vi "HRV_main.vi"() -> ()   [LabVIEW 2009]
uses:
  Instance           4 13Saved   HRV_3 .vi
  Instance           3 13Saved   HRV_3 .vi
  Instance           2 13Saved   HRV_3 .vi
  Instance           1 13Saved   HRV_3 .vi
  Instance           5 13Saved   HRV_3 .vi
  Instance           6 13Saved   HRV_3 .vi
  Instance           7 13Saved   HRV_3 .vi
  Instance           9 13Saved   HRV_3 .vi
  <vilib>/Analysis/5stat.llb/RMS (DBL).vi
  Instance          21 13Saved   HRV_3 .vi
  Instance          20 13Saved   HRV_3 .vi
  Instance          19 13Saved   HRV_3 .vi
  Instance          24 13Saved   HRV_3 .vi
  Instance          23 13Saved   HRV_3 .vi
  Instance          22 13Saved   HRV_3 .vi
  Instance          18 13Saved   HRV_3 .vi
  Instance          17 13Saved   HRV_3 .vi
  Instance          16 13Saved   HRV_3 .vi
  Instance          14 13Saved   HRV_3 .vi
  Instance          13 13Saved   HRV_3 .vi
  <vilib>/express/express analysis/Spectral/XNode/ExpressSpectralMeasurementsBlockNode.xnode
  <vilib>/express/express analysis/Spectral/Block/exnSpectralBlock spectral measurements PSD poly.vi
  <vilib>/express/express analysis/Spectral/Block/exnSpectralBlock spectral measurements PSD DDT.vi
  Instance          25 13Saved   HRV_3 .vi
  Instance          26 13Saved   HRV_3 .vi
  Instance          27 13Saved   HRV_3 .vi
  <vilib>/Utility/NIReport.llb/HTML Report Text Alignment.ctl
  <vilib>/Utility/NIReport.llb/NI_report.lvclass
  <vilib>/printing/OpenHTMLReport.llb/Open HTML Report in Browser (Refnum).vi
  <vilib>/Utility/NIReport.llb/Append Report Text (str wrap).vi
  <vilib>/Analysis/NI_AALPro.lvlib
  <vilib>/Analysis/NI_AALBase.lvlib
  <vilib>/Utility/NIReport.llb/NI_ReportGenerationCore.lvlib
panel:
  out "Waveform Graph":dynamicdata(graph)
  out "File Name:":string
  in  "Sample Rate:":sgl=500.034 min=1 max=20000 format="%.3g"
  in  "Tab Control 3":enum32{"RR-Intervals", "HRV"}(tab)=enum."HRV"
  in  "RR Rejection  Sensitivity :":dbl=0.5 min=0.0 max=1.0 format="%#.5g"
  in  "Resample Rate : (Hz):":dbl=2.0 format="%.3p"
  out "RR Waveforms":dbl[][](graph)
  out "HRV: Freq Domain":string[][](table)
  in  "HF2":dbl=0.4 caption="Begin Offset" min=0.0
  in  "HF1":dbl=0.15 caption="Begin Offset" min=0.0
  in  "LF2":dbl=0.15 caption="Begin Offset" min=0.0
  in  "LF1":dbl=0.04 caption="Begin Offset" min=0.0
  in  "TP 2":dbl=0.4 caption="Begin Offset" min=0.0
  in  "TP 1":dbl=0.04 caption="Begin Offset" min=0.0
  out "HRV: Time Domain":string[][](table)
  out "RR FFT 2":dynamicdata(graph) caption="Power Spectrum"
  out "ECG Waveform":dbl[][](graph)
  in  "Tab Control":enum32{"Controls", "Filters"}(tab)
  in  "File Type":u16(ring) items=["ASCII (*.txt)", "Binary (*.tdx)"]
  in  "Report Type":enum16{"Standard Report", "HTML"}(ring)=enum."HTML"
  in  "Save :":bool
  in  "Save RR data to file:":bool
  in  "Threshold:":dbl=1.0 step=0.001 format="%#.6f"
  out "Number of Peaks:":i32
  in  "Select ECG":bool
  in  "Report":bool
  in  "Bandstop":bool=TRUE
  in  "Lower Cut-Off":dbl=59.0 format="%#_4g"
  in  "Upper Cut-Off":dbl=61.0 format="%#_4g"
  in  "Bandpass":bool=TRUE
  in  "Upper Cut-Off":dbl=100.0 format="%#_4g"
  in  "Lower Cut-Off":dbl=0.05 format="%#_4g"
  # "Frequency Domain"
  # "Frequency Limits"
  # "LF Limits:"
  # "HF Limits:"
  # "Total Limits:"
  # "Time Domain"
  # "Bandpass"
  # "Bandstop"
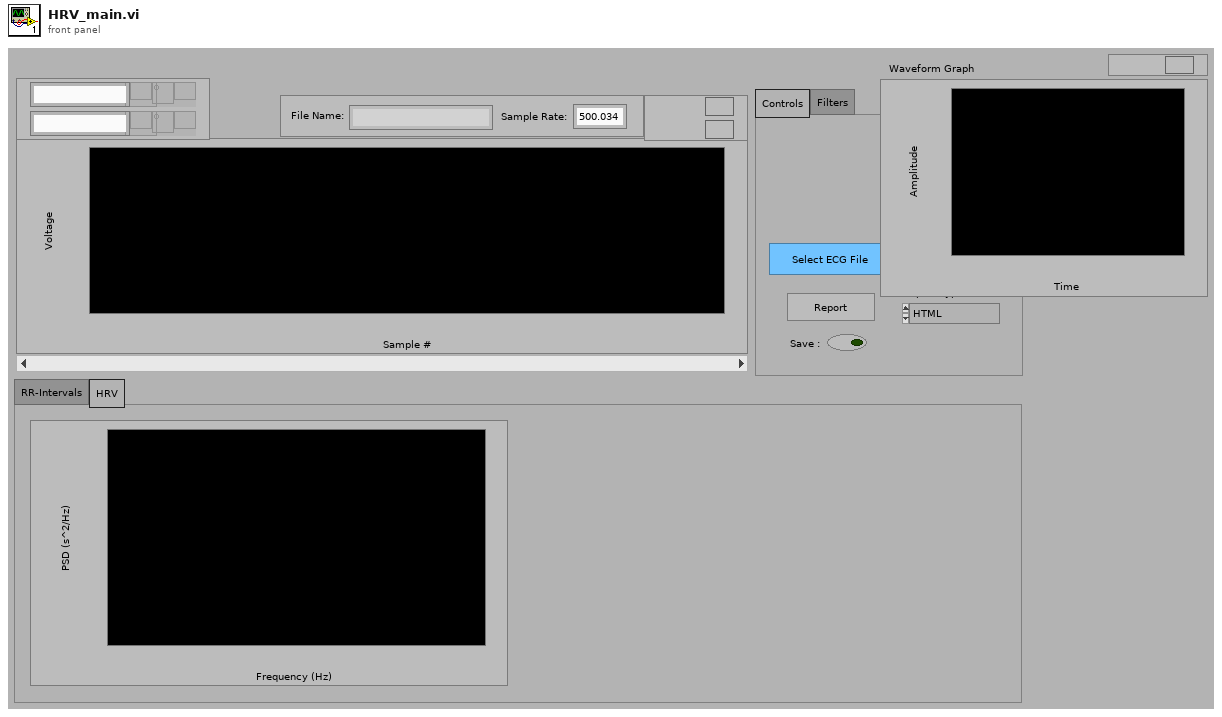
[diagram p1: front panel]
types:
  T1 = cluster{"averaging mode":u16, "weighting mode":u16, "number of averages":u32}
  T2 = cluster{"dB On (F)":bool, "unwrap phase (F)":bool, "convert to degree (F)":bool}
  T3 = typedef "NI_ReportGenerationCore.lvlib/HTML Report Text Alignment.ctl" = enum16{"(default)", "LEFT", "CENTER", "RIGHT"}
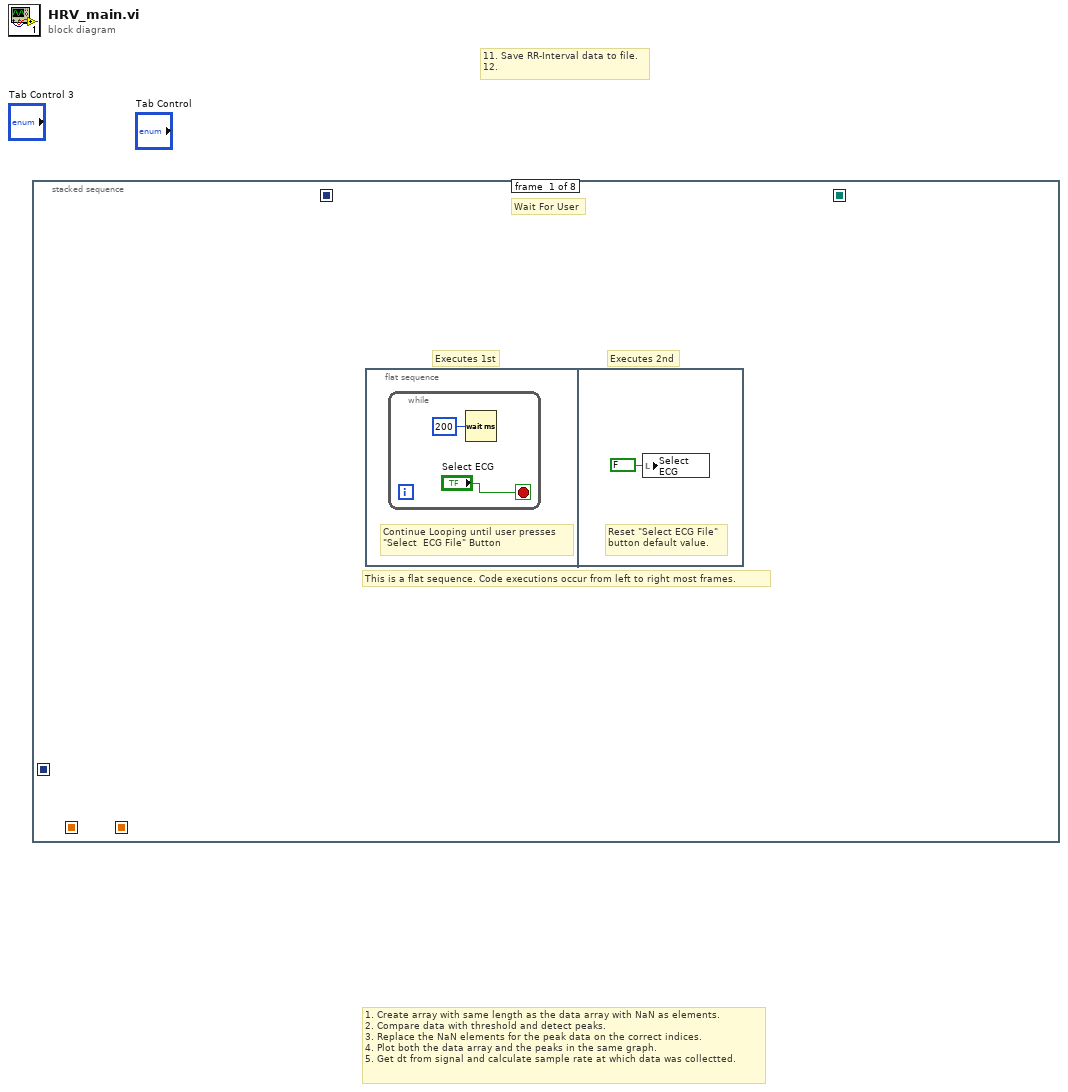
[diagram p0: block diagram]
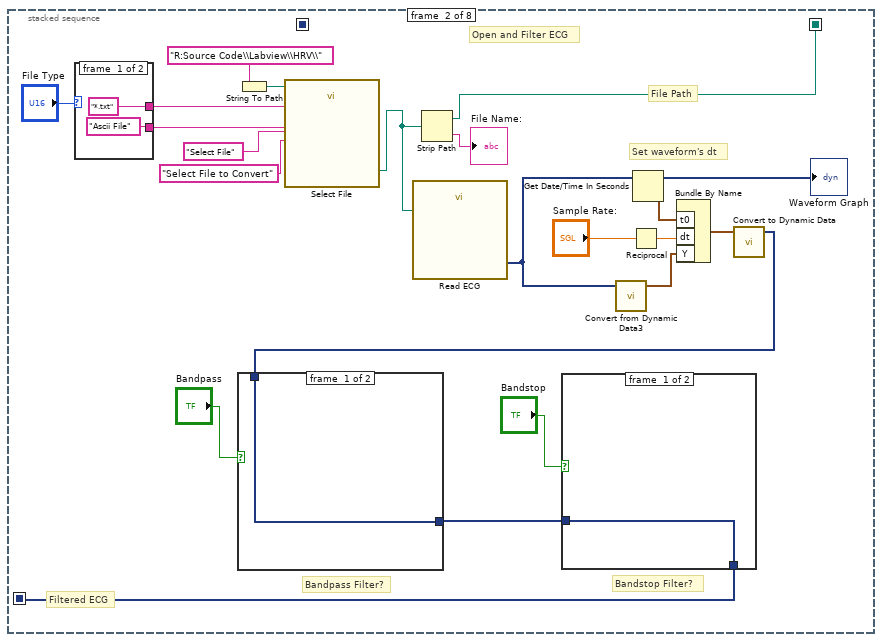
[diagram p2: hidden frame]
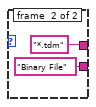
[diagram p3: hidden frame]
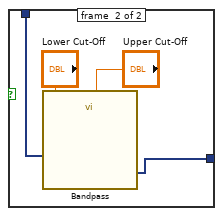
[diagram p4: hidden frame]
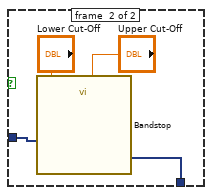
[diagram p5: hidden frame]
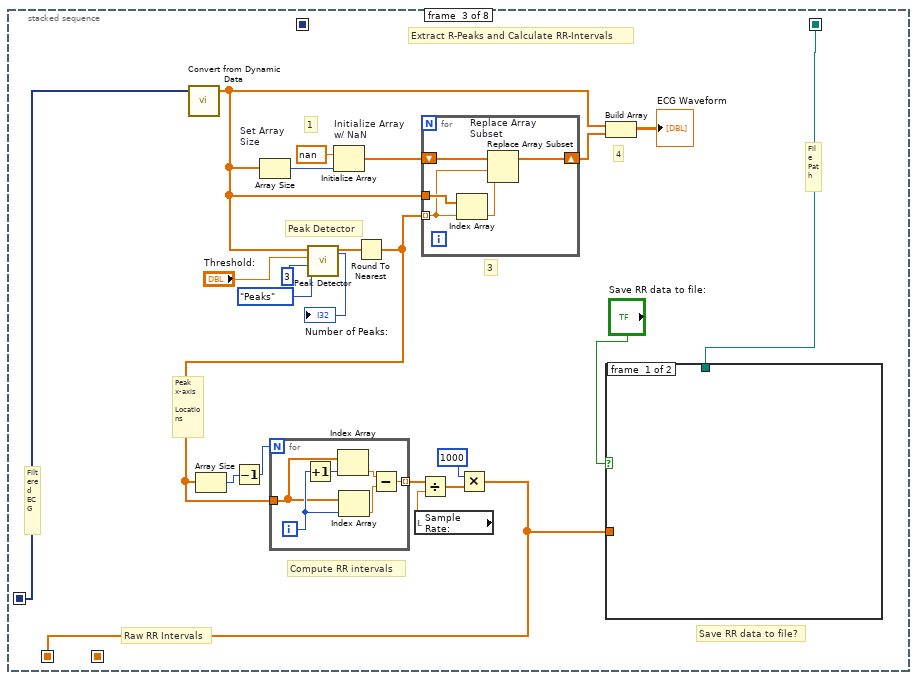
[diagram p6: hidden frame]
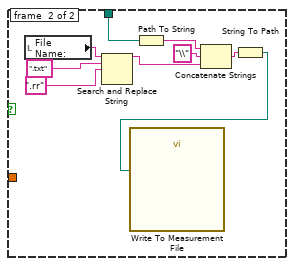
[diagram p7: hidden frame]
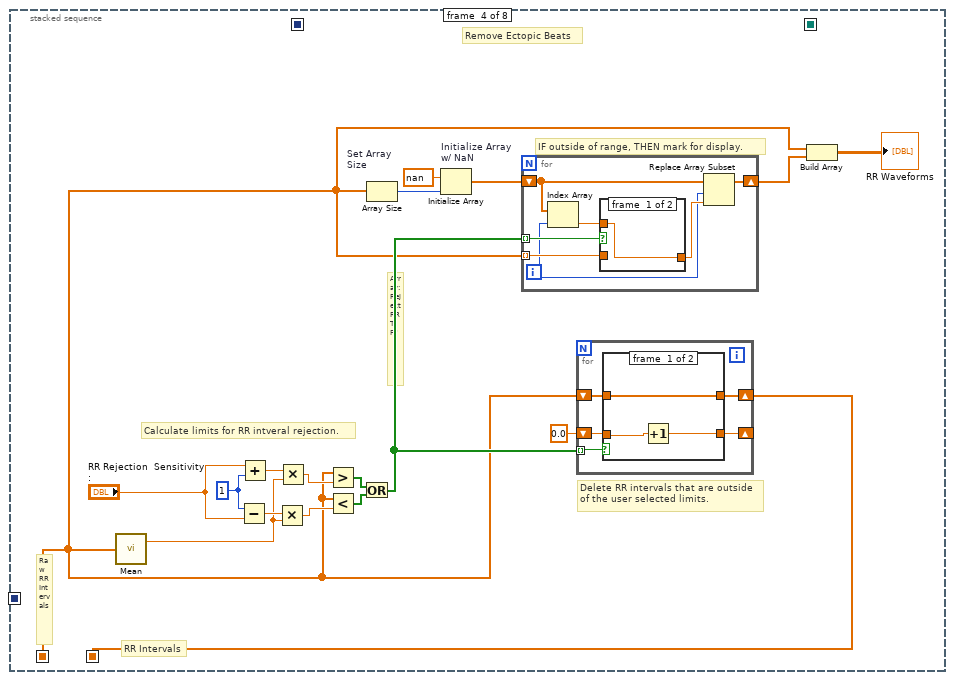
[diagram p8: hidden frame]
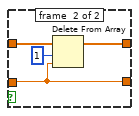
[diagram p9: hidden frame]
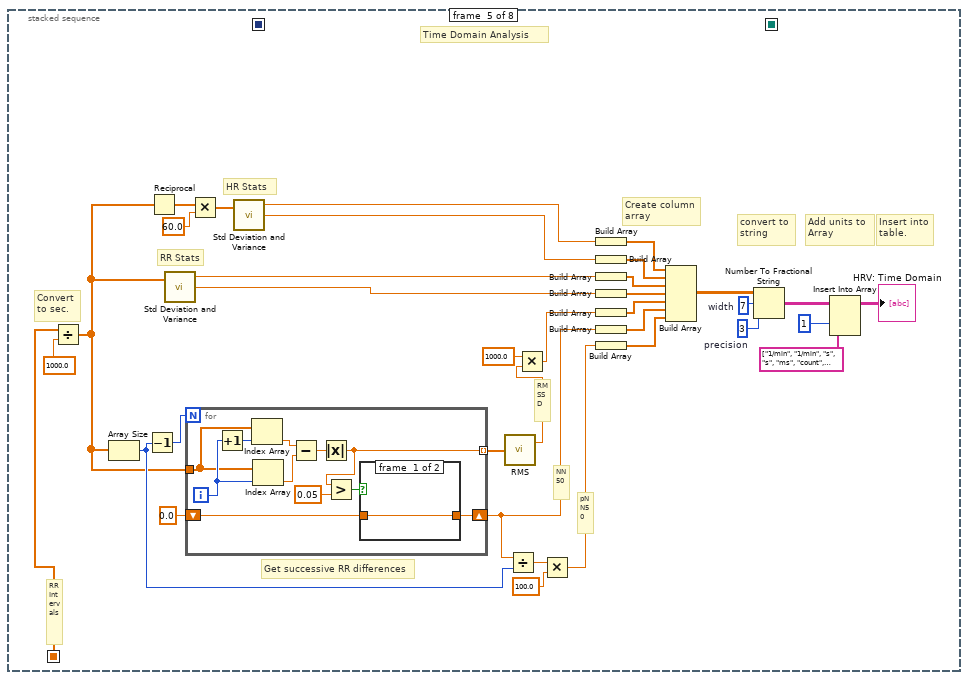
[diagram p11: hidden frame]
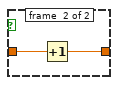
[diagram p12: hidden frame]
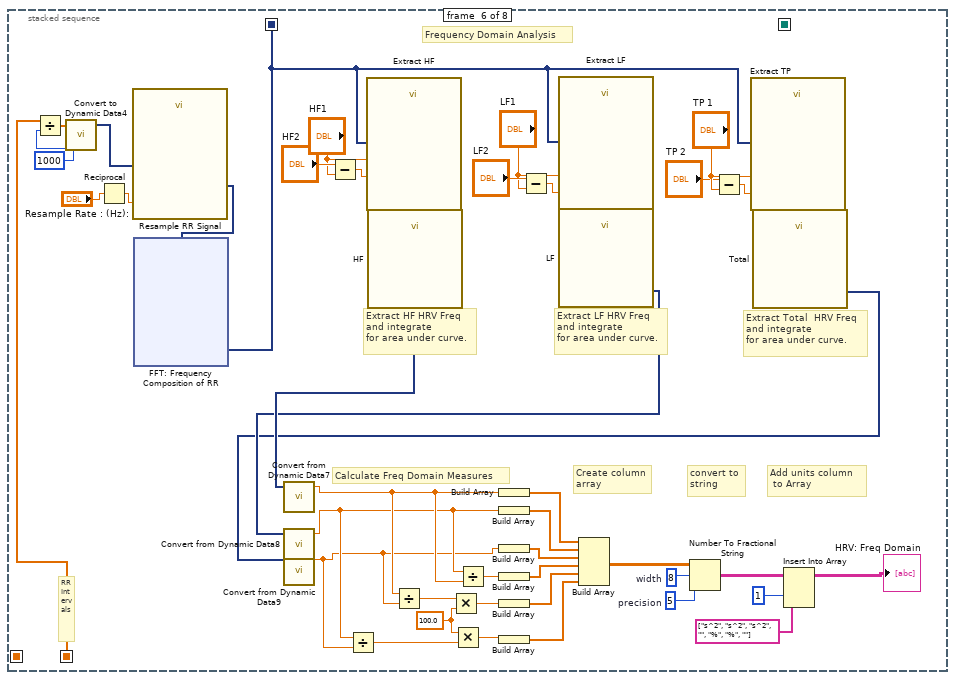
[diagram p13: hidden frame]
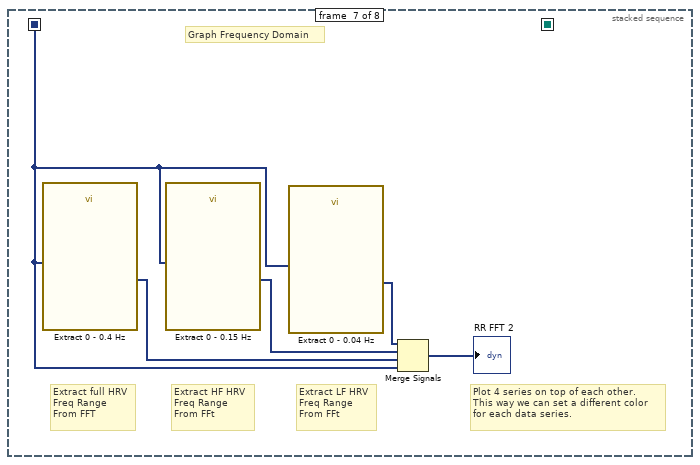
[diagram p14: hidden frame]
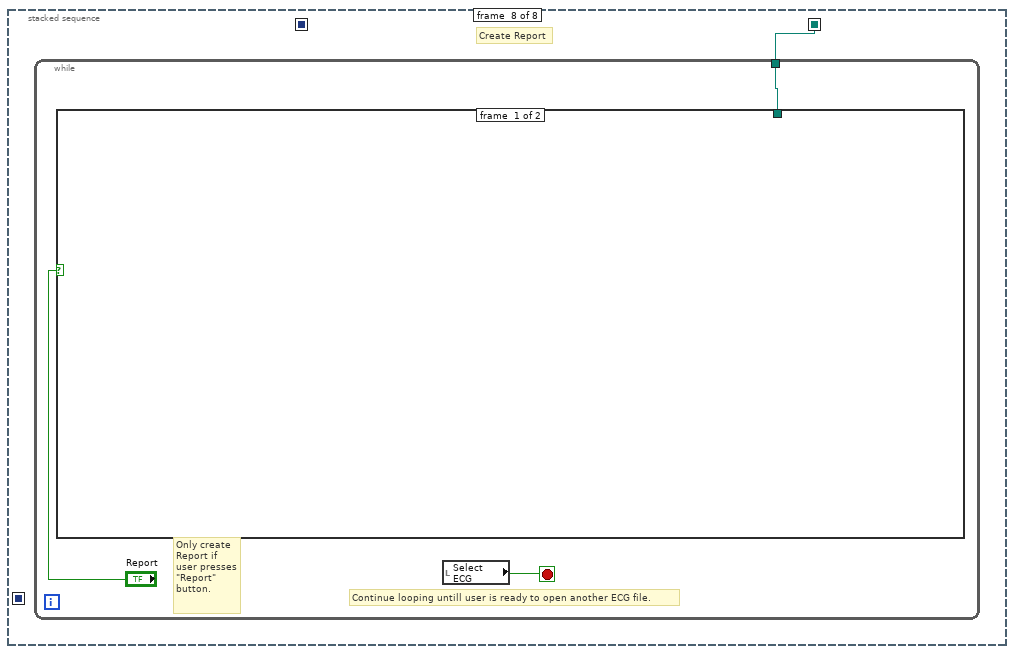
[diagram p15: hidden frame]
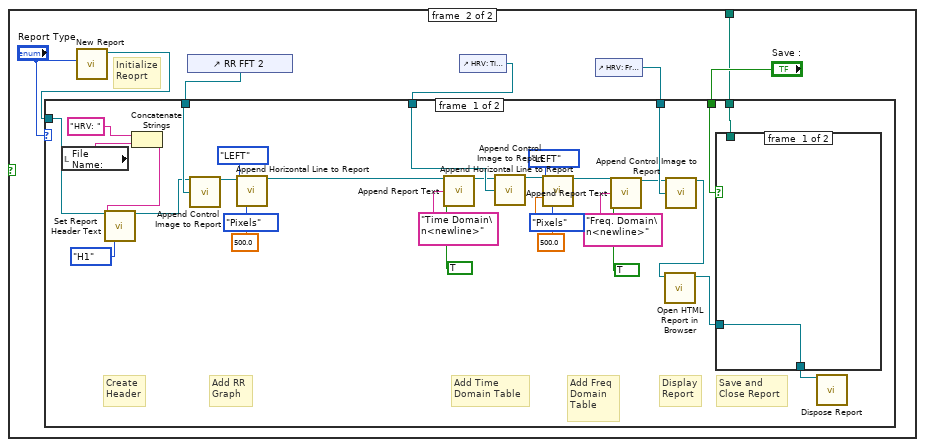
[diagram p16: hidden frame]
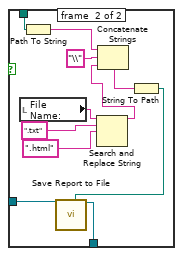
[diagram p17: hidden frame]
diagram:
  # "1. Create array with same length as the data array with NaN as elements.\n2. Compare data with threshold and detect peaks.\n3. Replace the NaN elements for the peak data on the correct indices.\n4. Plot both the data array and the peaks in the same graph.\n5. Get dt from signal and calculate sample rate at which data was collectted."
  # "11. Save RR-Interval data to file.\n12."
  n1 = stacked-sequence {
    seq-local: [_ w16 _ _ _ _ _ _] -> [_ _ w49 _ _ _ _ _]
    seq-local: [_ _ w41 _ _ _ _ _] -> [_ _ _ w84 _ _ _ _]
    seq-local: [_ w10 _ _ _ _ _ _] -> [_ _ w39 _ _ _ _ w228]
    seq-local: [_ _ _ _ _ w181 _ _] -> [_ _ _ _ _ _ w223 _]
    seq-local: [_ _ _ w82 _ _ _ _] -> [_ _ _ _ w120 w169 _ _]
    frame #0 {
      # "Executes 2nd"
      # "Executes 1st"
      # "This is a flat sequence. Code executions occur from left to right most frames."
      # "Wait For User"
      n2 = flat-sequence {
        frame #0 {
          # "Continue Looping until user presses\n\"Select  ECG File\" Button"
          n3 = while {
            stop <- "Select ECG" stop-if-true
            n4 = Wait (ms)(milliseconds to wait=u32 200) -> ()  [unwired: 1 out]
          }
        }
        frame #1 {
          # "Reset \"Select ECG File\"\nbutton default value."
          n5 = local write "Select ECG"(FALSE ("Select ECG")) -> ()
        }
      }
    }
    frame #1 {
      # "Filtered ECG"
      # "File Path"
      # "Set waveform's dt"
      # "Open and Filter ECG"
      # "Bandstop Filter?"
      # "Bandpass Filter?"
      n6 = case shown="1" "File Type" {
        tunnel: ["Ascii File" "Binary File"] -> w5
        tunnel: ["*.txt" "*.tdm"] -> w6
        frame #0 {
        }
        frame #1 {
        }
      }
      n7 = String To Path(string="R:Source Code\\Labview\\HRV\\") -> (path=w15:path)
      n8 = call "Select File"("start path"=w15, "prompt"="Select File to Convert", "button label"="Select File", "pattern (all files)"=w6, "pattern label"=w5) -> ("selected path"=w11:path)  [unwired: 7 in, 3 out]
      n9 = call "Read ECG"("File Name"=w11) -> ("Signals"=w4:dynamicdata)  [unwired: 5 in, 5 out]
      "Waveform Graph" <- w4
      n10 = Strip Path(path=w11) -> (stripped path=w10:path, name=→"File Name:":string)
      n11 = call "Convert from Dynamic Data3"("Dynamic Data Type"=w4) -> ("Waveform"=w23:waveform(dbl))  [unwired: 3 in]
      n12 = Reciprocal(x="Sample Rate:") -> (1/x=w22:sgl)
      n13 = Get Date/Time In Seconds() -> (seconds since 1Jan1904=w24:timestamp)
      n14 = Bundle By Name("t0"=w24, "dt"=w22, "Y"=w23) -> (w19:waveform(dbl))  [unwired: 1 in]
      n15 = call "Convert to Dynamic Data"("Waveform"=w19) -> ("Dynamic Data Type"=w18:dynamicdata)  [unwired: 3 in]
      n16 = case shown="True" "Bandpass" {
        tunnel: w18 -> [w29 w31]
        tunnel: [w29 w30] -> w17
        frame #0 {
        }
        frame #1 {
          n17 = call "Bandpass"("Lower Cut-Off"="Lower Cut-Off", "Upper Cut-Off"="Upper Cut-Off", "Signal"=w31) -> ("Filtered Signal"=w30:dynamicdata)  [unwired: 7 in, 1 out]
        }
      }
      n18 = case shown="True" "Bandstop" {
        tunnel: w17 -> [w34 w36]
        tunnel: [w34 w35] -> w16
        frame #0 {
        }
        frame #1 {
          n19 = call "Bandstop"("Lower Cut-Off"="Lower Cut-Off", "Upper Cut-Off"="Upper Cut-Off", "Signal"=w36) -> ("Filtered Signal"=w35:dynamicdata)  [unwired: 7 in, 1 out]
        }
      }
    }
    frame #2 {
      # "File Path"
      # "Peak Detector"
      # "Raw RR Intervals"
      # "Peak x-axis\n Locations"
      # "Save RR data to file?"
      # "Compute RR intervals"
      # "Filtered ECG"
      # "Extract R-Peaks and Calculate RR-Intervals"
      # "4"
      # "3"
      # "1"
      n20 = call "Convert from Dynamic Data"("Dynamic Data Type"=w49) -> ("Array"=w55:dbl[])  [unwired: 3 in]
      n21 = Array Size "Set Array\nSize"(array=w55) -> (size(s)=w59:i32)
      n22 = call <vilib>:"Peak Detector.vi"("peaks/valleys"=enum32{"Peaks", "Valleys"}."Peaks", "width"=3, "threshold"="Threshold:", "X"=w55) -> ("Locations"=w50:dbl[], "# found"=→"Number of Peaks:":i32)  [unwired: 3 in, 3 out]
      n23 = Initialize Array "Initialize Array\nw/ NaN"(nan, w59) -> (w58:dbl[])
      n24 = Round To Nearest(number=w50) -> (nearest integer value=w40:dbl[])
      n25 = Array Size(array=w40) -> (size(s)=w48:i32)
      n26 = Decrement(x=w48) -> (x-1=w46:i32)
      n27 = for {
        N: w46 -> [_]
        tunnel: w40 -> [w71]
        tunnel: [w70] -> w47 mode=indexing
        i -> [w72]
        n28 = Increment(x=w72) -> (x+1=w75:i32)
        n29 = Index Array(array=w71, index=w75) -> (element=w74:dbl)
        n30 = Index Array(array=w71, index=w72) -> (element=w73:dbl)
        n31 = Subtract(x=w74, y=w73) -> (x-y=w70:dbl)
      }
      n32 = local read "Sample Rate:"() -> (w42:sgl)
      n33 = Divide(x=w47, y=w42) -> (x/y=w43:dbl[])
      n34 = for {
        tunnel: w40 -> [w77] mode=indexing
        shift-right: [w79] -> w57
        shift-left: w58 -> [w80]
        tunnel: w55 -> [w78]
        n35 = Index Array "Index Array"(array=w78, index=w77) -> (element=w76:dbl)
        n36 = Replace Array Subset "Replace Array\nSubset"(array=w80, new element=w76, index=w77) -> (w79:dbl[])
      }
      n37 = Multiply(x=1000, y=w43) -> (x*y=w41:dbl[])
      n38 = Build Array "Build Array"(w55, w57) -> (→"ECG Waveform":dbl[][])
      n39 = case shown="True" "Save RR data to file:" {
        tunnel: w41 -> [_ _]
        tunnel: w39 -> [_ w62]
        frame #0 {
        }
        frame #1 {
          n40 = local read "File Name:"() -> (w68:string)
          n41 = Search and Replace String(input string=w68, search string=".txt", replace string=".rr" ("search string")) -> (result string=w64:string)  [unwired: 5 in, 3 out]
          n42 = Path To String(path=w62) -> (string=w69:string)
          n43 = Concatenate Strings(w69, "\\" ("string"), w64) -> (w65:string)
          n44 = String To Path(string=w65) -> (path=w61:path)
          n45 = call "Write To Measurement File"("File Name"=w61) -> ()  [unwired: 8 in, 3 out]
        }
      }
    }
    frame #3 {
      w98 = 1
      # "Remove Ectopic Beats"
      # "IF outside of range, THEN mark for display."
      # "Delete RR intervals that are outside\nof the user selected limits."
      # "RR Intervals"
      # "Array: Reject RR T/F?"
      # "Calculate limits for RR intveral rejection."
      # "Raw RR Intervals"
      n46 = call <vilib>:"Mean.vi"("X"=w84) -> ("mean"=w94:dbl)  [unwired: 1 out]
      n47 = Subtract(x=w98, y="RR Rejection  Sensitivity :") -> (x-y=w95:dbl)
      n48 = Add(x="RR Rejection  Sensitivity :", y=w98) -> (x+y=w96:dbl)
      n49 = Multiply(x=w95, y=w94) -> (x*y=w86:dbl)
      n50 = Multiply(x=w96, y=w94) -> (x*y=w87:dbl)
      n51 = Greater?(x=w84, y=w87) -> (0:w89:bool[])
      n52 = Less?(x=w84, y=w86) -> (x < y?=w88:bool[])
      n53 = Or(x=w89, y=w88) -> (x .or. y?=w85:bool[])
      n54 = Array Size "Set Array\nSize"(array=w84) -> (size(s)=w92:i32)
      n55 = Initialize Array "Initialize Array\nw/ NaN"(nan, w92) -> (w91:dbl[])
      n56 = for {
        shift-right: [w117] -> w90
        shift-left: w91 -> [w116]
        tunnel: w85 -> [w115] mode=indexing
        tunnel: w84 -> [w113] mode=indexing
        i -> [w111]
        n57 = Index Array(array=w116, index=w111) -> (element=w114:dbl)
        n58 = case shown="False" w115 {
          tunnel: w114 -> [w118 _]
          tunnel: w113 -> [_ w119]
          tunnel: [w118 w119] -> w112
          frame #0 {
          }
          frame #1 {
          }
        }
        n59 = Replace Array Subset(array=w116, new element=w112, index=w111) -> (w117:dbl[])
      }
      n60 = for {
        tunnel: w85 -> [w101] mode=indexing
        shift-right: [w102] -> w82
        shift-left: w84 -> [w103]
        shift-right: [w99] -> _
        shift-left: 0.0 -> [w100]
        n61 = case shown="True" w101 {
          tunnel: w103 -> [w106 w110]
          tunnel: [w106 w108] -> w102
          tunnel: w100 -> [w105 w107]
          tunnel: [w104 w107] -> w99
          frame #0 {
            n62 = Increment(x=w105) -> (x+1=w104:dbl)
          }
          frame #1 {
            n63 = Delete From Array(array=w110, length=1, index=w107) -> (array with subset deleted=w108:dbl[])  [unwired: 1 out]
          }
        }
      }
      n64 = Build Array "Build Array"(w84, w90) -> (→"RR Waveforms":dbl[][])
    }
    frame #4 {
      w153 = 3  # precision
      w154 = 7  # width
      # "Convert\nto sec."
      # "RR Intervals"
      # "Insert into\ntable."
      # "Add units to\nArray"
      # "convert to\nstring"
      # "Create column array"
      # "pNN50"
      # "NN50"
      # "RMSSD"
      # "RR Stats"
      # "HR Stats"
      # "Get successive RR differences"
      # "Time Domain Analysis"
      n65 = Divide(x=w120, y=1000.0) -> (x/y=w126:dbl[])
      n66 = Array Size(array=w126) -> (size(s)=w130:i32)
      n67 = Decrement(x=w130) -> (x-1=w121:i32)
      n68 = Reciprocal(x=w126) -> (1/x=w139:dbl[])
      n69 = call <vilib>:"Std Deviation and Variance.vi"("X"=w126) -> ("mean"=w134:dbl, "standard deviation"=w133:dbl)  [unwired: 1 in, 1 out]
      n70 = for {
        N: w121 -> [_]
        tunnel: w126 -> [w161]
        tunnel: [w155] -> w132 mode=indexing
        shift-right: [w157] -> w131
        shift-left: 0.0 -> [w158]
        i -> [w162]
        n71 = Increment(x=w162) -> (x+1=w165:i32)
        n72 = Index Array(array=w161, index=w165) -> (element=w164:dbl)
        n73 = Index Array(array=w161, index=w162) -> (element=w163:dbl)
        n74 = Subtract(x=w164, y=w163) -> (x-y=w156:dbl)
        n75 = Absolute Value(x=w156) -> (abs(x)=w155:dbl)
        n76 = Greater?(x=w155, y=0.05) -> (0:w159:bool)
        n77 = case shown="True" w159 {
          tunnel: w158 -> [w166 w168]
          tunnel: [w166 w167] -> w157
          frame #0 {
          }
          frame #1 {
            n78 = Increment(x=w168) -> (x+1=w167:dbl)
          }
        }
      }
      n79 = Multiply(x=w139, y=60.0) -> (x*y=w137:dbl[])
      n80 = call <vilib>:"Std Deviation and Variance.vi"("X"=w137) -> ("mean"=w136:dbl, "standard deviation"=w135:dbl)  [unwired: 1 in, 1 out]
      n81 = call-poly <vilib>:"RMS.vi"("X"=w132) -> ("rms value"=w124:dbl)  [unwired: 1 out]
      n82 = Divide(x=w131, y=w130) -> (x/y=w129:dbl)
      n83 = Multiply(x=1000.0 ("y"), y=w124) -> (x*y=w123:dbl)
      n84 = Multiply(x=w129, y=100.0) -> (x*y=w127:dbl)
      n85 = Build Array(w136) -> (w150:dbl[])
      n86 = Build Array(w135) -> (w144:dbl[])
      n87 = Build Array(w134) -> (w145:dbl[])
      n88 = Build Array(w133) -> (w146:dbl[])
      n89 = Build Array(w123) -> (w147:dbl[])
      n90 = Build Array(w131) -> (w148:dbl[])
      n91 = Build Array(w127) -> (w149:dbl[])
      n92 = Build Array(w150, w144, w145, w146, w147, w148, w149) -> (w142:dbl[][])
      n93 = Number To Fractional String(number=w142, width (-)=w154, precision (6)=w153) -> (F-format string=w143:string[][])  [unwired: 1 in]
      n94 = Insert Into Array(array=w143, index (col)=1 ("disabled index (col)"), new element=string[] ["1/min", "1/min", "s", "s", "ms", "count", "%"] ("new element/subarray")) -> (→"HRV: Time Domain":string[][])  [unwired: 1 in]
    }
    frame #5 {
      w178 = 100.0 ("y")
      w200 = 5  # precision
      w201 = 8  # width
      # "Calculate Freq Domain Measures"
      # "RR Intervals"
      # "Extract Total  HRV Freq\nand integrate\nfor area under curve."
      # "Extract LF HRV Freq\nand integrate\nfor area under curve."
      # "Extract HF HRV Freq\nand integrate\nfor area under curve."
      # "Add units column\n to Array"
      # "convert to\nstring"
      # "Create column array"
      # "Frequency Domain Analysis"
      n95 = Divide(x=w169, y=1000) -> (x/y=w172:dbl[])
      n96 = call "Convert to Dynamic Data4"("Array"=w172) -> ("Dynamic Data Type"=w174:dynamicdata)  [unwired: 3 in]
      n97 = Reciprocal(x="Resample Rate : (Hz):") -> (1/x=w175:dbl)
      n98 = call "Resample RR Signal"("dt"=w175, "Signals"=w174) -> ("Resampled Signals"=w170:dynamicdata)  [unwired: 7 in, 2 out]
      n99 = xnode "FFT: Frequency Composition of RR"("Signals"=w170) -> ("PSD"=w181:dynamicdata)  [unwired: 1 in, 1 out]
      n100 = Subtract(x="HF2", y="HF1") -> (x-y=w203:dbl)
      n101 = call "Extract HF"("Length"=w203, "Begin Offset"="HF1", "Signals"=w181) -> ("Section"=w213:dynamicdata)  [unwired: 7 in, 1 out]
      n102 = call "HF"("Signals"=w213) -> ("Result"=w188:dynamicdata)  [unwired: 5 in, 1 out]
      n103 = call "Convert from Dynamic Data7"("Dynamic Data Type"=w188) -> ("Scalar"=w184:dbl)  [unwired: 3 in]
      n104 = Build Array(w184) -> (w197:dbl[])
      n105 = Subtract(x="LF2", y="LF1") -> (x-y=w205:dbl)
      n106 = call "Extract LF"("Length"=w205, "Begin Offset"="LF1", "Signals"=w181) -> ("Section"=w212:dynamicdata)  [unwired: 7 in, 1 out]
      n107 = call "LF"("Signals"=w212) -> ("Result"=w187:dynamicdata)  [unwired: 5 in, 1 out]
      n108 = call "Convert from Dynamic Data8"("Dynamic Data Type"=w187) -> ("Scalar"=w183:dbl)  [unwired: 3 in]
      n109 = Divide(x=w183, y=w184) -> (x/y=w185:dbl)
      n110 = Build Array(w183) -> (w192:dbl[])
      n111 = Build Array(w185) -> (w194:dbl[])
      n112 = Subtract(x="TP 2", y="TP 1") -> (x-y=w210:dbl)
      n113 = call "Extract TP"("Length"=w210, "Begin Offset"="TP 1", "Signals"=w181) -> ("Section"=w211:dynamicdata)  [unwired: 7 in, 1 out]
      n114 = call "Total"("Signals"=w211) -> ("Result"=w186:dynamicdata)  [unwired: 5 in, 1 out]
      n115 = call "Convert from Dynamic Data9"("Dynamic Data Type"=w186) -> ("Scalar"=w182:dbl)  [unwired: 3 in]
      n116 = Divide(x=w183, y=w182) -> (x/y=w177:dbl)
      n117 = Divide(x=w184, y=w182) -> (x/y=w180:dbl)
      n118 = Multiply(x=w180, y=w178) -> (x*y=w179:dbl)
      n119 = Multiply(x=w178, y=w177) -> (x*y=w176:dbl)
      n120 = Build Array(w182) -> (w193:dbl[])
      n121 = Build Array(w179) -> (w195:dbl[])
      n122 = Build Array(w176) -> (w196:dbl[])
      n123 = Build Array(w197, w192, w193, w194, w195, w196) -> (w190:dbl[][])
      n124 = Number To Fractional String(number=w190, width (-)=w201, precision (6)=w200) -> (F-format string=w191:string[][])  [unwired: 1 in]
      n125 = Insert Into Array(array=w191, index (col)=1 ("disabled index (col)"), new element=string[] ["s^2", "s^2", "s^2", "", "%", "%", ""] ("new element/subarray")) -> (→"HRV: Freq Domain":string[][])  [unwired: 1 in]
    }
    frame #6 {
      # "Plot 4 series on top of each other.\nThis way we can set a different color\nfor each data series."
      # "Extract LF HRV\nFreq Range\nFrom FFt"
      # "Extract HF HRV\nFreq Range\nFrom FFt"
      # "Extract full HRV\nFreq Range\nFrom FFT"
      # "Graph Frequency Domain"
      n126 = call "Extract 0 - 0.4 Hz"("Signals"=w223) -> ("Section"=w225:dynamicdata)  [unwired: 9 in, 1 out]
      n127 = call "Extract 0 - 0.15 Hz"("Signals"=w223) -> ("Section"=w226:dynamicdata)  [unwired: 9 in, 1 out]
      n128 = call "Extract 0 - 0.04 Hz"("Signals"=w223) -> ("Section"=w227:dynamicdata)  [unwired: 9 in, 1 out]
      n129 = Merge Signals(w227, w226, w225, w223) -> (→"RR FFT 2":dynamicdata)
    }
    frame #7 {
      # "Create Report"
      n130 = while {
        tunnel: w228 -> [w230]
        stop <- w229 stop-if-true
        # "Continue looping untill user is ready to open another ECG file."
        # "Only create\nReport if\nuser presses\n\"Report\"\nbutton."
        n131 = case shown="True" "Report" {
          tunnel: w230 -> [_ w232]
          frame #0 {
          }
          frame #1 {
            # "Initialize\nReoprt"
            n132 = call <vilib>:"New Report.vi"("report type"="Report Type") -> ("report out"=w238:refnum<class "NI_report.lvclass">)  [unwired: 13 in, 1 out]
            n133 = control-ref of="RR FFT 2"() -> (w236:refnum<vi>)
            n134 = control-ref of="HRV: Time Domain"() -> (w234:refnum<vi>)
            n135 = control-ref of="HRV: Freq Domain"() -> (w233:refnum<vi>)
            n136 = case shown="\"HTML\"" "Report Type" {
              tunnel: w238 -> [w266 _]
              tunnel: "Save :" -> [w267 _]
              tunnel: w236 -> [w265 _]
              tunnel: w234 -> [w262 _]
              tunnel: w233 -> [w255 _]
              tunnel: w232 -> [w243 _]
              frame #0 {
                # "Display\nReport"
                # "Add Freq\nDomain\nTable"
                # "Add Time\nDomain Table"
                # "Add RR\nGraph"
                # "Create\nHeader"
                # "Save and\nClose Report"
                n137 = local read "File Name:"() -> (w246:string)
                n138 = Concatenate Strings("HRV: " ("left header text"), w246) -> (w244:string)
                n139 = call-dynamic "Set Report Header Text.vi"("report in"=w266, "left header text"=w244, "HTML header size"=enum16{"H1", "H2", "H3", "H4", "H5", "H6", "H7"}."H1") -> ("report out"=w245:refnum<class "NI_report.lvclass">)  [unwired: 11 in, 1 out]
                n140 = call-dynamic "Append Control Image to Report.vi"("report in"=w245, "ctrl reference"=w265) -> ("report out"=w261:refnum<class "NI_report.lvclass">)  [unwired: 10 in, 3 out]
                n141 = call-dynamic "Append Horizontal Line to Report.vi"("report in"=w261, "align (default)"=HTML_Report_Text_Alignment."LEFT", "width (100=default)"=500.0 ("width (0=default)"), "width units"=enum16{"Pixels", "Percentage"}."Pixels") -> ("report out"=w239:refnum<class "NI_report.lvclass">)  [unwired: 10 in, 1 out]
                n142 = call-poly <vilib>:"Append Report Text.vi"("report in"=w239, "text"="Time Domain\n<newline>", "append on new line? (F)"=TRUE) -> ("report out"=w257:refnum<class "NI_report.lvclass">)  [unwired: 9 in, 3 out]
                n143 = call-dynamic "Append Control Image to Report.vi"("report in"=w257, "ctrl reference"=w262) -> ("report out"=w256:refnum<class "NI_report.lvclass">)  [unwired: 10 in, 3 out]
                n144 = call-dynamic "Append Horizontal Line to Report.vi"("report in"=w256, "align (default)"=HTML_Report_Text_Alignment."LEFT", "width (100=default)"=500.0 ("width (0=default)"), "width units"=enum16{"Pixels", "Percentage"}."Pixels") -> ("report out"=w252:refnum<class "NI_report.lvclass">)  [unwired: 10 in, 1 out]
                n145 = call-poly <vilib>:"Append Report Text.vi"("report in"=w252, "text"="Freq. Domain\n<newline>", "append on new line? (F)"=TRUE) -> ("report out"=w251:refnum<class "NI_report.lvclass">)  [unwired: 9 in, 3 out]
                n146 = call-dynamic "Append Control Image to Report.vi"("report in"=w251, "ctrl reference"=w255) -> ("report out"=w242:refnum<class "NI_report.lvclass">)  [unwired: 10 in, 3 out]
                n147 = call-poly <vilib>:"Open HTML Report in Browser.vi"("report in"=w242) -> ("report out"=w240:refnum<class "NI_report.lvclass">)  [unwired: 12 in, 2 out]
                n148 = case shown="True" w267 {
                  tunnel: w243 -> [_ w278]
                  tunnel: w240 -> [w269 w273]
                  tunnel: [w269 w272] -> w241
                  frame #0 {
                  }
                  frame #1 {
                    n149 = local read "File Name:"() -> (w275:string)
                    n150 = Path To String(path=w278) -> (string=w279:string)
                    n151 = Search and Replace String(input string=w275, search string=".txt", replace string=".html" ("search string")) -> (result string=w270:string)  [unwired: 5 in, 3 out]
                    n152 = Concatenate Strings(w279, "\\" ("string"), w270) -> (w280:string)
                    n153 = String To Path(string=w280) -> (path=w274:path)
                    n154 = call-dynamic "Save Report to File.vi"("report in"=w273, "report file path"=w274) -> ("report out"=w272:refnum<class "NI_report.lvclass">)  [unwired: 12 in, 1 out]
                  }
                }
                n155 = call-dynamic "Dispose Report.vi"("report in"=w241) -> ()  [unwired: 14 in, 1 out]
              }
              frame #1 {
              }
            }
          }
        }
        n156 = local read "Select ECG"() -> (w229:bool)
      }
    }
  }
